vi "Vision Research Phantom Series PhCon PhGetPartitions.vi"(0 "CN in":u32=1, 2 "pCount":u32=1, 5 "Error In (no error)":errorcluster) -> (14 "CN out":u32=1, 16 "pCount out":u32=1, 17 "pPartitionSize":u32[](array[numeric]), 19 "Error Out":errorcluster)   [LabVIEW 2013, in "VRI.lvlib"]
doc: "PhCon.dll\n\nPhGetPartitions\nHRESULT PhGetPartitions(UINT CN, PUINT pCount, PUINT pPartitionSize);\n\nParameters Description\nCN (in) Camera number.\npCount (in, out) pPartitionSize array size at input & count of partitions \n at output.\npPartitionSize (out) Array of the memory size allocated to each partition\nReturn HRESULT (0=Ok)\nComments Provide the sizes (megabytes) of partitions defined \n in the camera (v7)\n\nWritten by:\nBLOOMY CONTROLS, INC\nWINDSOR, CT 06095, USA\n860-298-9925\nwww.bloomy.com\nV1.0.0\nMay, 2004"
uses:
  VRI.lvlib
  Phantom DLLs/PhCon.dll
panel:
  # "For instructions on the use of this VI, press Ctrl+H to display the help window and move the mouse over the icon, controls, and indicators"
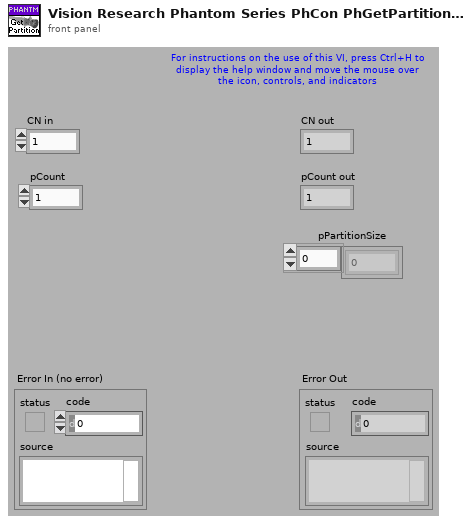
[diagram p1: front panel]
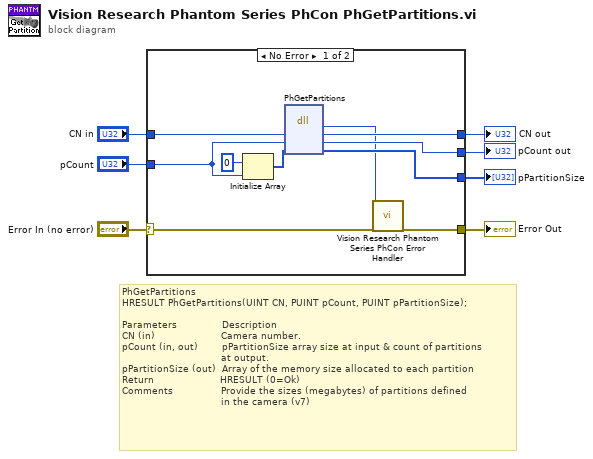
[diagram p0: block diagram]
diagram:
  # "PhGetPartitions\nHRESULT PhGetPartitions(UINT CN, PUINT pCount, PUINT pPartitionSize);\n\nParameters               Description\nCN (in)                      Camera number.\npCount (in, out)        pPartitionSize array size at input & count of partitions \n                                 at output.\npPartitionSize (out)  Array of the memory size allocated to each partition\nReturn                      HRESULT (0=Ok)\nComments                Provide the sizes (megabytes) of partitions defined \n                                 in the camera (v7)"
  n1 = case shown="No Error" "Error In (no error)" {
    selector: "Error In (no error)" -> [w17 w19]
    tunnel: [w16 w19] -> w6
    tunnel: "CN in" -> [w15 w18]
    tunnel: [w14 w18] -> w4
    tunnel: [w13 _] -> w3
    tunnel: [w12 _] -> w2
    tunnel: "pCount" -> [w11 _]
    frame No Error {
      n2 = Initialize Array(u32 0 ("element"), w11) -> (w8:u32[])
      n3 = dll-call lib="C:/Projects/SDK/32-bit/Vision Research Phantom Series Labview Driver/Phantom DLLs/PhCon.dll" fn="PhGetPartitions"("CN"=w15, "pCount"=w11, "pPartitionSize"=w8) -> ("HRESULT"=w10:i32, "CN"=w14:u32, "pCount"=w12:u32, "pPartitionSize"=w13:u32[])  [unwired: 3 in, 2 out]
      n4 = call "Vision Research Phantom Series PhCon Error Handler.vi"("ErrNo"=w10, "Error In (no error)"=w17) -> ("Error Out"=w16:errorcluster)  [unwired: 17 out]
    }
    frame Error {
    }
  }
  "Error Out" <- w6
  "CN out" <- w4
  "pPartitionSize" <- w3
  "pCount out" <- w2
